vi "GUI_PL1-FlowCheck.vi"() -> ()   [LabVIEW 2013]
uses:
  shared programs/GUI_Template/GUI_master/tcp_new_data_event.ctl
  shared programs/GUI_Template/GUI_master/tcp new data cluster.ctl
panel:
  out "Pressure::2":dbl caption="Pressure" min=0.0 max=100.0
  out "Flow::2":dbl caption="Flow" min=0.0 max=0.0
  in  "GUIdevice 2":string="BELLA_LowPressureControl"
  in  "Limit":dbl=4.0 min=-10.0 max=10.0
  out "XY Graph":cluster{dbl[], dbl[]}[](graph)
  in  "Clear":bool
  out "DeltaFlow::1":dbl caption="DeltaFlow" min=-10.0 max=10.0
  in  "GUIdevice 1":string="PL1-FlowCheck"
  in  "stop":bool
  out "tcp data event":T1
  out "error IO 2":errorcluster
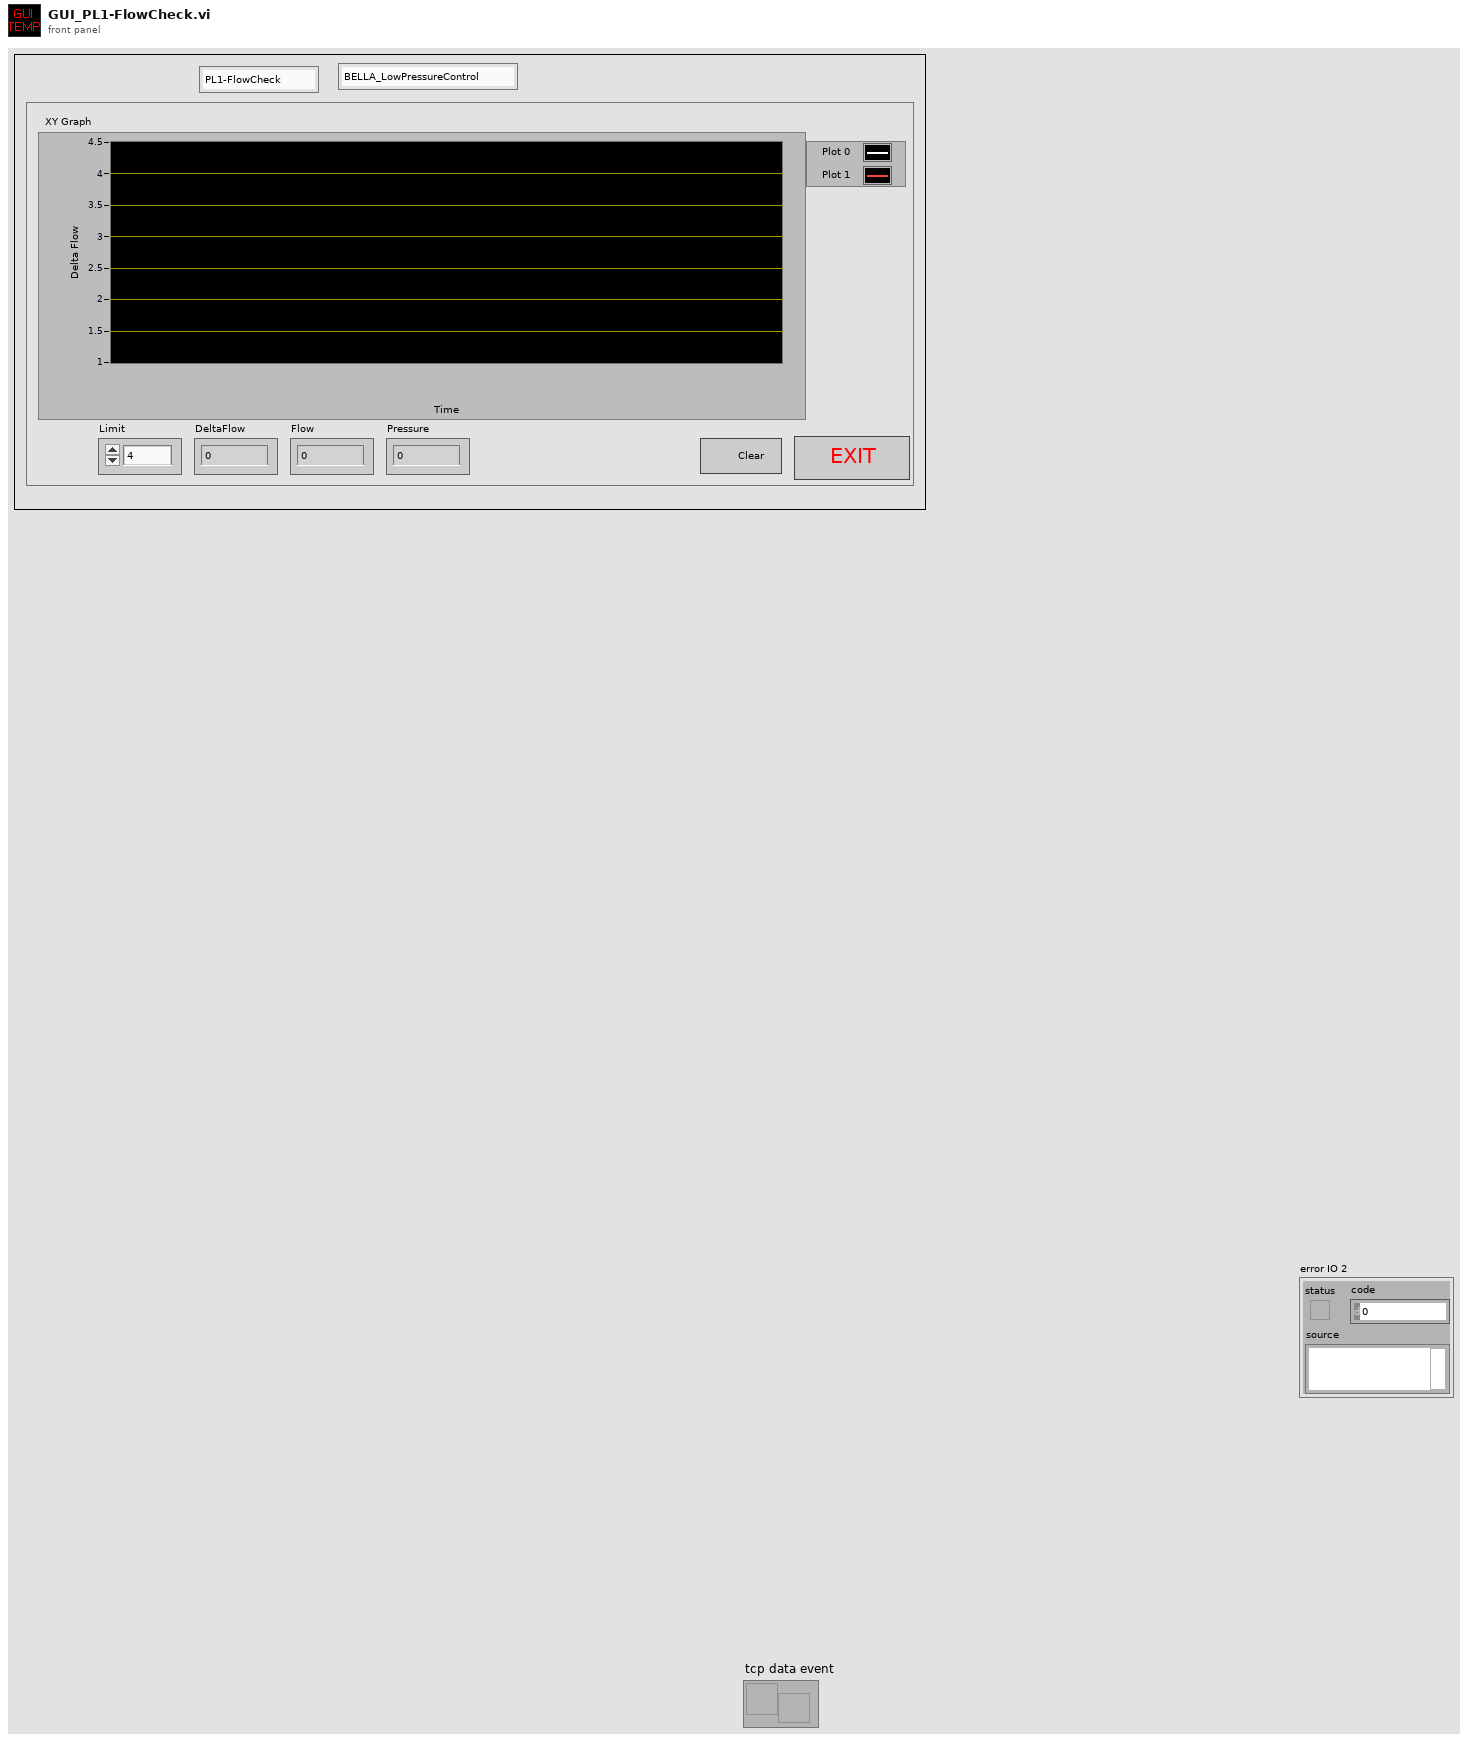
[diagram p1: front panel]
types:
  T1 = typedef "tcp_new_data_event.ctl" = refnum<user-event>
  T2 = typedef "tcp new data cluster.ctl" = cluster{"EventEnum":enum16{"new data", "connection status update"}, "Device name":string}
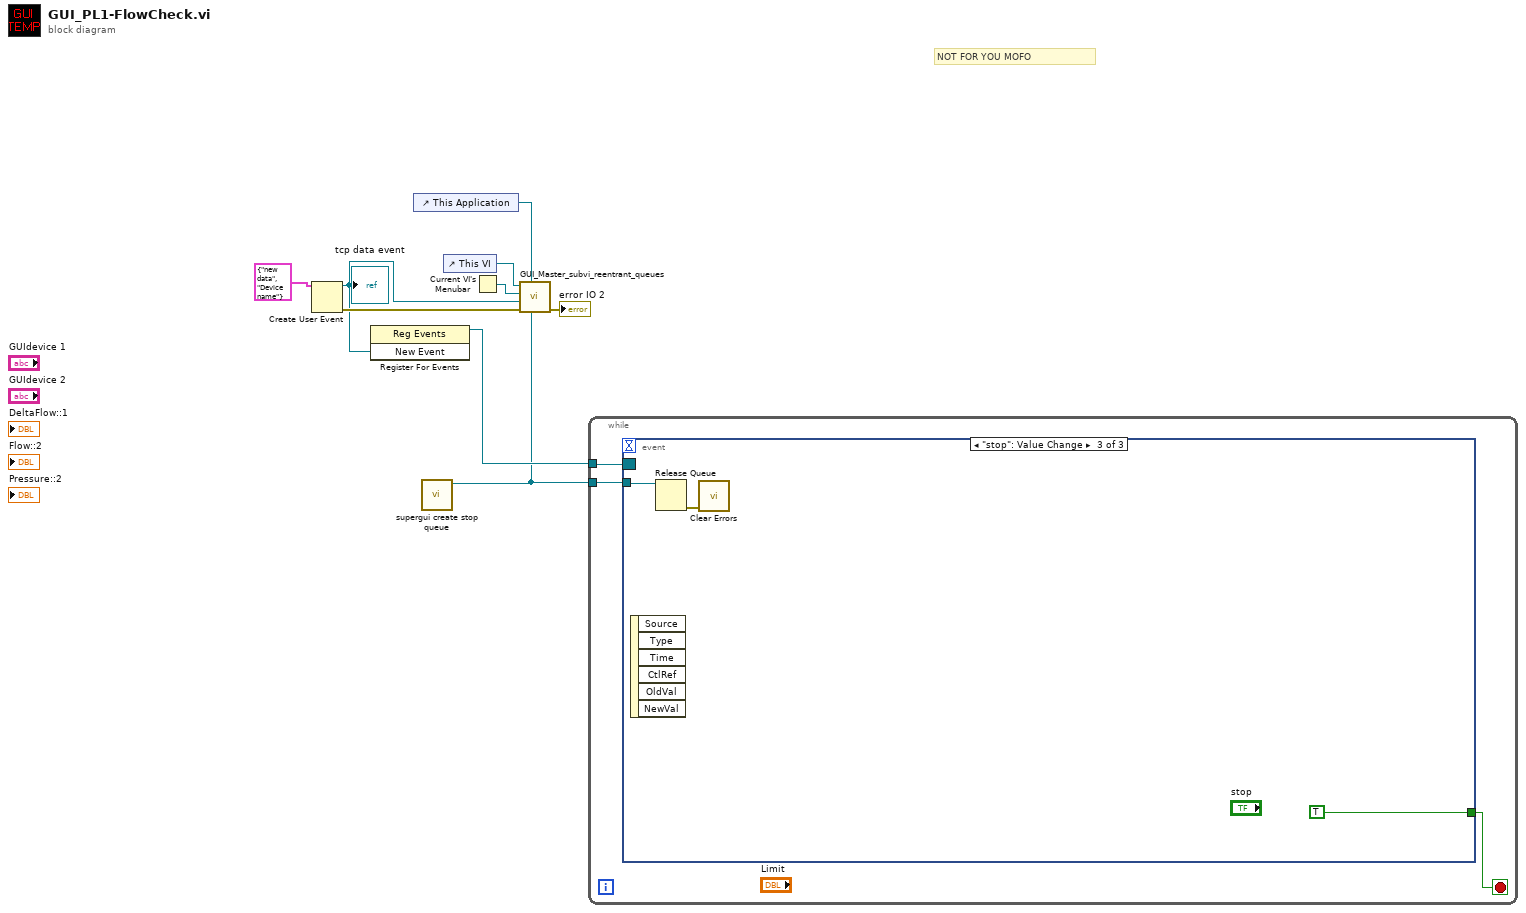
[diagram p0: block diagram]
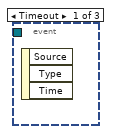
[diagram p2: hidden frame]
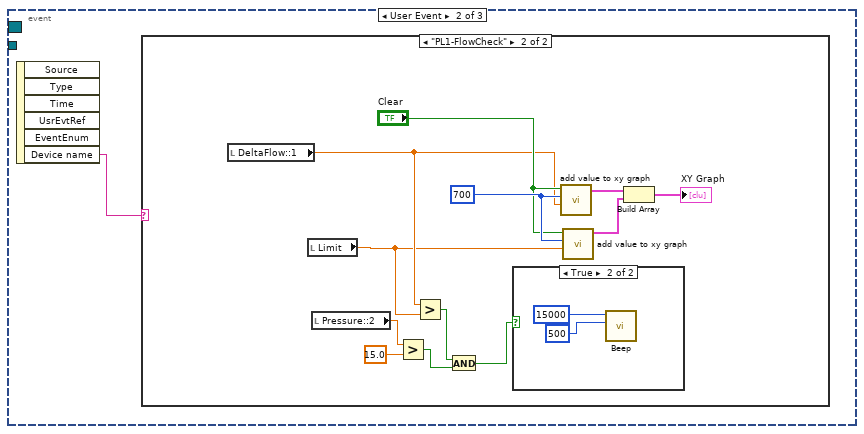
[diagram p3: hidden frame]
diagram:
  # "NOT FOR YOU MOFO"
  n1 = Create User Event(user event datatype=T2 {"EventEnum"=enum."new data", "Device name"="Device name"} ("New Event")) -> (user event=w4:refnum<user-event>, error out=w5:errorcluster)  [unwired: 1 in]
  "tcp data event" <- w4
  n2 = register-events(w4) -> (reference out=w2:refnum<event-registration>)  [unwired: 2 in, 1 out]
  n3 = control-ref of="This Application"() -> (w3:refnum<vi>)
  n4 = call "supergui create stop queue.vi"() -> ("STOP Queue out"=w1:refnum<queue>)  [unwired: 11 in]
  n5 = control-ref of="This VI"() -> (w8:refnum<vi>)
  n6 = Current VI's Menubar() -> (w7:refnum<k9>)
  n7 = call "GUI_Master_subvi_reentrant_queues.vi"("STOP Queue in"=w1, "This Application"=w3, "error in (no error)"=w5, "tcp data event"=w4, "Caller menu reference"=w7, "Caller VI ref"=w8) -> ("error out"=→"error IO 2":errorcluster)  [unwired: 5 in]
  n8 = while {
    tunnel: w2 -> [w12]
    tunnel: w1 -> [w10]
    stop <- w11 stop-if-true
    n9 = event shown="[2] \"stop\": Value Change" {
      selector: w12 -> [_ _ _]
      dyn-events: _ -> [_ _ _]
      timeout: _ -> [_ _ _]
      tunnel: [_ _ TRUE ("stop")] -> w11
      tunnel: w10 -> [_ _ w29]
      event Timeout {
        n10 = event-data() -> ()  [unwired: 1 in, 3 out]
      }
      event User Event {
        n11 = event-data() -> ("Device name"=w13:string)  [unwired: 1 in, 5 out]
        n12 = case shown="\"PL1-FlowCheck\"" w13 {
          frame "False", Default {
          }
          frame "PL1-FlowCheck" {
            w25 = 700 ("max points")
            n13 = local read "DeltaFlow::1"() -> (w20:dbl)
            n14 = local read "Limit"() -> (w19:dbl)
            n15 = local read "Pressure::2"() -> (w18:dbl)
            n16 = Greater?(x=w18, y=15.0) -> (0:w15:bool)
            n17 = Greater?(x=w20, y=w19) -> (0:w16:bool)
            n18 = And(x=w16, y=w15) -> (x .and. y?=w14:bool)
            n19 = case shown="True" w14 {
              frame False {
              }
              frame True {
                n20 = call <vilib>:"Beep.vi"("duration (msec)"=u32 500, "frequency (Hz)"=u32 15000) -> ()  [unwired: 10 in]
              }
            }
            n21 = call "add value to xy graph.vi"("new value"=w20, "max points"=w25, "Wire in Stop To Clear Graph on Each Run"="Clear") -> ("XY Graph"=w23:cluster{dbl[], dbl[]})  [unwired: 8 in]
            n22 = call "add value to xy graph.vi"("new value"=w19, "max points"=w25, "Wire in Stop To Clear Graph on Each Run"="Clear") -> ("XY Graph"=w22:cluster{dbl[], dbl[]})  [unwired: 8 in]
            n23 = Build Array(w23, w22) -> (→"XY Graph":cluster{dbl[], dbl[]}[])
          }
        }
      }
      event "stop": Value Change {
        n24 = event-data() -> ()  [unwired: 1 in, 6 out]
        n25 = Release Queue(queue=w29) -> (error out=w28:errorcluster)  [unwired: 2 in, 2 out]
        n26 = call <vilib>:"Clear Errors.vi"("error in (no error)"=w28) -> ()  [unwired: 6 in, 1 out]
      }
    }
  }
